vi "Get X-Point Foci.vi"(1 "Chromosome Length":i32, 2 "X-Point Type":T1) -> (0 "X-Points":i32[](array[numeric]))   [LabVIEW 2016, in "N-Point Crossover.lvclass"]
uses:
  N-Point Crossover.lvclass
  _Typedefs/X-Point Crossover.ctl
panel:
  # "INPUTS"
  # "OUTPUTS"
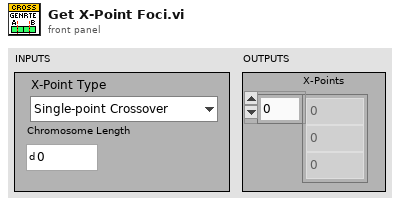
[diagram p1: front panel]
types:
  T1 = typedef "N-Point Crossover.lvclass/X-Point Crossover.ctl" = enum16{"Single-point Crossover", "Dual-point Crossover"}
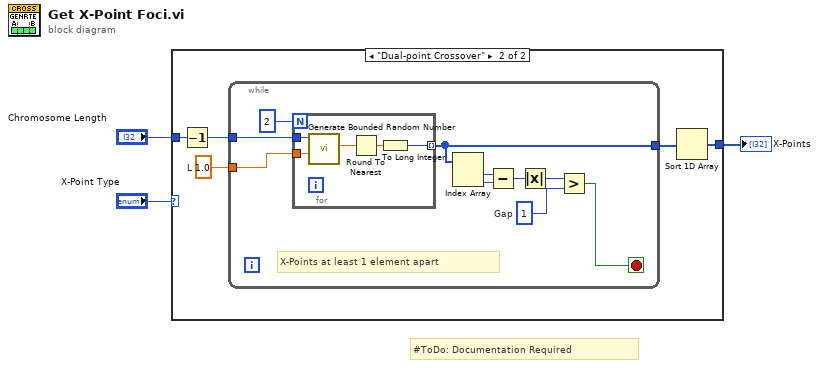
[diagram p0: block diagram]
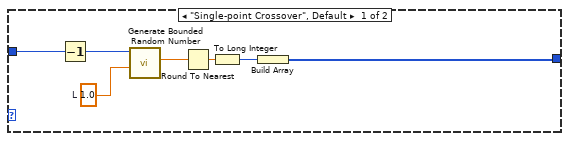
[diagram p2: hidden frame]
diagram:
  # "#ToDo: Documentation Required"
  n1 = case shown="\"Dual-point Crossover\"" "X-Point Type" {
    tunnel: "Chromosome Length" -> [w9 w13]
    tunnel: [w5 w12] -> w1
    frame "Single-point Crossover", Default {
      w10 = 1.0  # L
      n2 = Decrement(x=w9) -> (x-1=w8:i32)
      n3 = call "Generate Bounded Random Number.vi"("Lower (0.00)"=w10, "Upper (1.00)"=w8) -> ("Random Number"=w7:dbl)  [unwired: 9 in]
      n4 = Round To Nearest(number=w7) -> (nearest integer value=w6:dbl)
      n5 = To Long Integer(number=w6) -> (32bit integer=w4:i32)
      n6 = Build Array(w4) -> (w5:i32[])
    }
    frame "Dual-point Crossover" {
      w15 = 1.0  # L
      n7 = Decrement(x=w13) -> (x-1=w14:i32)
      n8 = while {
        tunnel: w15 -> [w25]
        tunnel: w14 -> [w24]
        tunnel: [w17] -> w11
        stop <- w16 stop-if-true
        w18 = 1  # Gap
        # "X-Points at least 1 element apart"
        n9 = for {
          N: 2 -> [_]
          tunnel: w25 -> [w30]
          tunnel: w24 -> [w29]
          tunnel: [w26] -> w17 mode=indexing
          n10 = call "Generate Bounded Random Number.vi"("Lower (0.00)"=w30, "Upper (1.00)"=w29) -> ("Random Number"=w28:dbl)  [unwired: 9 in]
          n11 = Round To Nearest(number=w28) -> (nearest integer value=w27:dbl)
          n12 = To Long Integer(number=w27) -> (32bit integer=w26:i32)
        }
        n13 = Index Array(array=w17) -> (element #1=w22:i32, element #2=w21:i32)  [unwired: 2 in]
        n14 = Subtract(x=w22, y=w21) -> (x-y=w20:i32)
        n15 = Absolute Value(x=w20) -> (abs(x)=w19:i32)
        n16 = Greater?(x=w19, y=w18) -> (0:w16:bool)
      }
      n17 = Sort 1D Array(array=w11) -> (sorted array=w12:i32[])
    }
  }
  "X-Points" <- w1
